vi "PlotUncert.vi"(7 "ePhases":T1) -> (11 "Plot Out":cluster{dbl, "Time":dbl, dbl[][]}(graph))   [LabVIEW 2014]
uses:
  typedefs/ePhases.ctl
panel:
  in  "Plot In":cluster{dbl, "Time":dbl, dbl[][]}[](array[cluster])
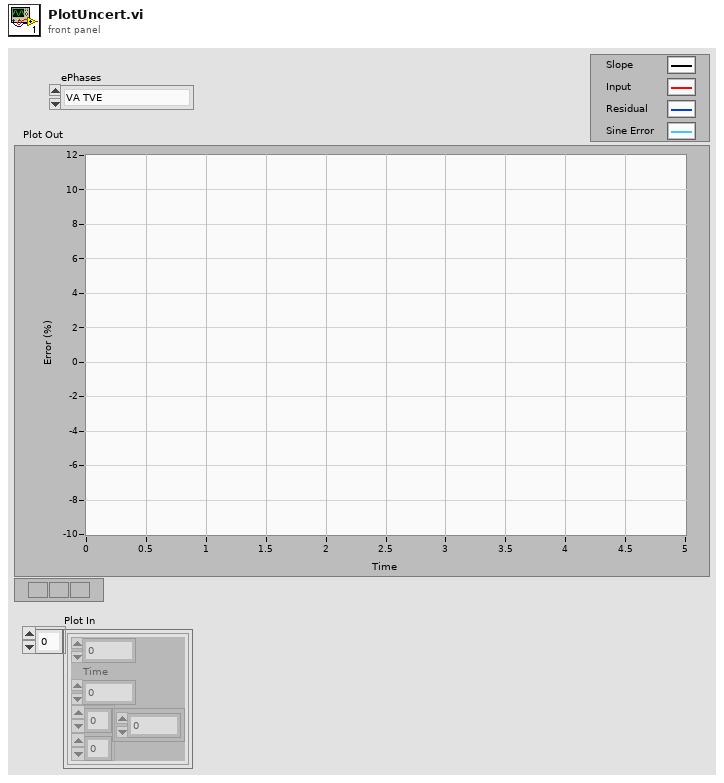
[diagram p1: front panel]
types:
  T1 = typedef "ePhases.ctl" = enum16{"VA TVE", "VA Mag ", "VA Phase", "VB TVE", "VB Mag", "VB Phase", "VC TVE", "VC Mag", "VC Phase", "V+ TVE", "V+ Mag", "V+ Phase", "IA TVE", "IA Mag", "IA Phase", "IB TVE", "IB Mag", "IB Phase", "IC TVE", "IC Mag", "IC Phase", "I+ TVE", "I+ Mag", "I+ Phase", "FE", "RFE"}
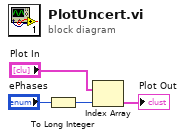
[diagram p0: block diagram]
diagram:
  n1 = To Long Integer(number="ePhases") -> (32bit integer=w4:i32)
  n2 = Index Array(array="Plot In", index=w4) -> (element=→"Plot Out":cluster{dbl, "Time":dbl, dbl[][]})
